vi "checkBegin.vi"(8 "error in (no error)":errorcluster, 10 "Game":refnum<class "Game.lvclass">, 11 "NormalDefensiveWithDuelistPlay in":refnum<class "NormalDefensiveWithDuelistPlay.lvclass">) -> (0 "error out":errorcluster, 2 "Duelist?":bool, 3 "NormalDefensiveWithDuelistPlay out":refnum<class "NormalDefensiveWithDuelistPlay.lvclass">)   [LabVIEW 2018, in "NormalDefensiveWithDuelistPlay.lvclass"]
uses:
  NormalDefensiveWithDuelistPlay.lvclass
  Game_class/Game.lvclass
  Events_class/Events.lvclass
  Utilities_class/Utilities.lvclass
  Events_class/Events.lvclass/Events.ctl
  Game_class/Game.lvclass/Game.ctl
  Ball_class/Ball.lvclass/Ball.ctl
  Object_class/Object.lvclass/Object.ctl
  Events_class/Read ball_inside_our_goalie_area.vi
  Game_class/Read Parameters.lvclass.vi
  Game_class/Read OffensiveTeam.vi
  Game_class/Read BallRef.vi
  Game_class/Read FieldRef.vi
  Ball_class/Read v_x.vi
  Ball_class/Read v_y.vi
  Object_class/Read x.vi
  Object_class/Read y.vi
  Ball_class/Ball.lvclass
  C:/Users/Ronaldo/Desktop/Phoenix/SSL_AI/Object_class/Object.lvclass
  Field_class/Field.lvclass
  Parameters_class/Parameters.lvclass
  Ally_class/Ally.lvclass
panel:
  in  "Events":refnum<class "Events.lvclass">
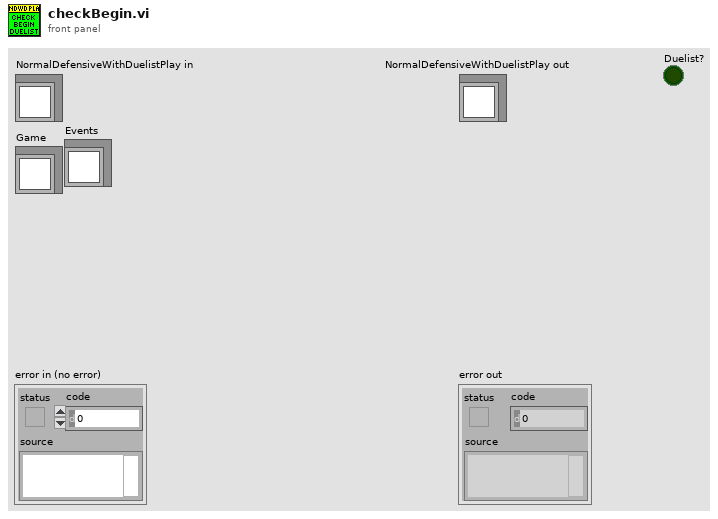
[diagram p1: front panel]
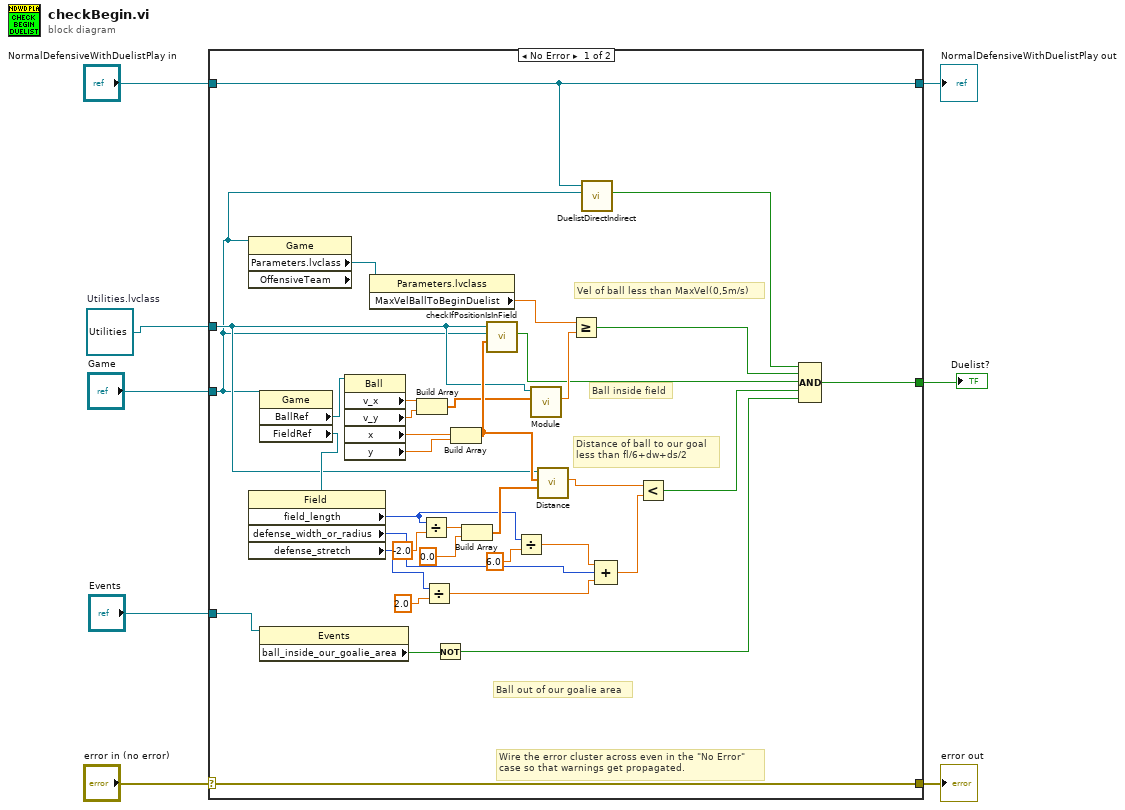
[diagram p0: block diagram]
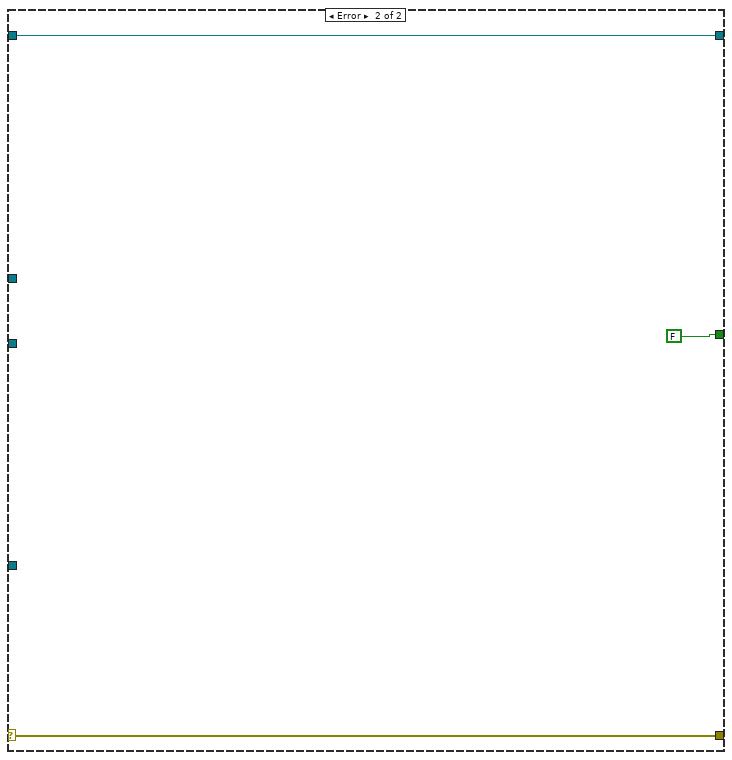
[diagram p2: hidden frame]
diagram:
  w4 = refnum<class "Utilities.lvclass"> refnum  # Utilities.lvclass
  n1 = case shown="No Error" "error in (no error)" {
    selector: "error in (no error)" -> [w44 w47]
    tunnel: [w44 w47] -> w7
    tunnel: [w11 w46] -> w5
    tunnel: "NormalDefensiveWithDuelistPlay in" -> [w11 w46]
    tunnel: w4 -> [w17 _]
    tunnel: "Game" -> [w10 _]
    tunnel: "Events" -> [w40 _]
    tunnel: [w12 FALSE] -> w1
    frame No Error {
      # "Vel of ball less than MaxVel(0,5m/s)"
      # "Ball inside field"
      # "Distance of ball to our goal\nless than fl/6+dw+ds/2"
      # "Ball out of our goalie area"
      # "Wire the error cluster across even in the \"No Error\"\ncase so that warnings get propagated."
      n2 = property class="Game" props=["Parameters.lvclass", "OffensiveTeam"](reference=w10) -> ("Parameters.lvclass"=w23:refnum<class "Parameters.lvclass">)  [unwired: 1 in, 3 out]
      n3 = property class="Game"(reference=w10) -> ("BallRef"=w43:refnum<class "Ball.lvclass">, "FieldRef"=w38:refnum<class "Field.lvclass">)  [unwired: 1 in, 2 out]
      n4 = property class="Field"(reference=w38) -> ("field_length"=w32:i32, "defense_width_or_radius"=w27:i32, "defense_stretch"=w30:i32)  [unwired: 1 in, 2 out]
      n5 = property class="Events"(reference=w40) -> ("ball_inside_our_goalie_area"=w39:bool)  [unwired: 1 in, 2 out]
      n6 = property class="Ball"(reference=w43) -> ("v_x"=w22:dbl, "v_y"=w21:dbl, "x"=w42:dbl, "y"=w41:dbl)  [unwired: 1 in, 2 out]
      n7 = property class="Parameters.lvclass"(reference=w23) -> ("MaxVelBallToBeginDuelist"=w20:dbl)  [unwired: 1 in, 2 out]
      n8 = Build Array(w22, w21) -> (w19:dbl[])
      n9 = Divide(x=w32, y=-2.0) -> (x/y=w36:dbl)
      n10 = Divide(x=w30, y=2.0) -> (x/y=w26:dbl)
      n11 = Not(x=w39) -> (.not. x?=w13:bool)
      n12 = Build Array(w42, w41) -> (w34:dbl[])
      n13 = Build Array(w36, 0.0) -> (w33:dbl[])
      n14 = call "checkIfPositionIsInField.vi"("Position"=w34, "Game"=w10, "Utilities in"=w17) -> ("Position Is In Field?"=w15:bool)  [unwired: 6 in, 2 out]
      n15 = Divide(x=w32, y=6.0) -> (x/y=w28:dbl)
      n16 = call-dynamic "Module.vi"("2D vector"=w19, "Utilities in"=w17) -> ("Modulo"=w18:dbl)  [unwired: 7 in, 2 out]
      n17 = call-dynamic "Distance.vi"("P1"=w33, "P2"=w34, "Utilities in"=w17) -> ("Distance"=w25:dbl)  [unwired: 6 in, 2 out]
      n18 = Greater Or Equal?(x=w20, y=w18) -> (x >= y?=w16:bool)
      n19 = call-dynamic "DuelistDirectIndirect.vi"("Game in"=w10, "NormalDefensiveWithDuelistPlay in"=w11) -> ("duelist ?"=w9:bool)  [unwired: 7 in, 2 out]
      n20 = Compound Arithmetic op=ADD(w28, w27, w26) -> (w24:dbl)
      n21 = Less?(x=w25, y=w24) -> (x < y?=w14:bool)
      n22 = Compound Arithmetic op=AND(w9, w16, w15, w14, w13) -> (w12:bool)
    }
    frame Error {
    }
  }
  "error out" <- w7
  "NormalDefensiveWithDuelistPlay out" <- w5
  "Duelist?" <- w1
